vi "Main Page.vi"(8 "error in (no error)":errorcluster, 11 "Node Ptr":T1 format="%.0x") -> (0 "error out":errorcluster)   [LabVIEW 2016, in "FPGA Addon System Explorer.lvlib"]
uses:
  FPGA Addon System Explorer.lvlib
  <vilib>/NI Veristand/Custom Device API/Custom Device Item Ref.ctl
  Shared/FG Action.ctl
  <vilib>/NI/NI VeriStand Hardware Discovery/Types/Filter Type.ctl
  Shared/Constants.vi
  <vilib>/NI Veristand/Custom Device API/NI VeriStand - Get Item Property.vi
  <vilib>/NI Veristand/Custom Device API/Get Item Property (Path).vi
  <vilib>/NI Veristand/Custom Device API/Get Item Property (String).vi
  <vilib>/NI Veristand/Custom Device API/NI VeriStand - Set Item Property.vi
  <vilib>/NI Veristand/Custom Device API/Set Item Property (Path).vi
  <vilib>/NI Veristand/Custom Device API/Set Item Property (String).vi
  <vilib>/NI VeriStand/Custom Device API/Custom Device API.lvlib
  Shared/FPGA Addon Shared.lvlib
  <vilib>/NI/NI VeriStand Hardware Discovery/NIVS Hardware Discovery.lvlib
  VeriStand-FPGA-Resource-Manager/Source/FPGA Resource Manager System Definition.lvlib
panel:
  in  "RIO Browse":bool
  out "Version":string
  in  "SHDocVw.IWebBrowser":refnum<k7>(container)
  in  "RIO Device":string
  in  "Bitfile path":path
  in  "Header 2":cluster{"Section Name":string}={"Section Name"="Custom Device Item Settings"}
  in  "Header":cluster{"Section Name":string}={"Section Name"="Custom Device Item Settings"}
  in  "Description":string
  in  "Name":string
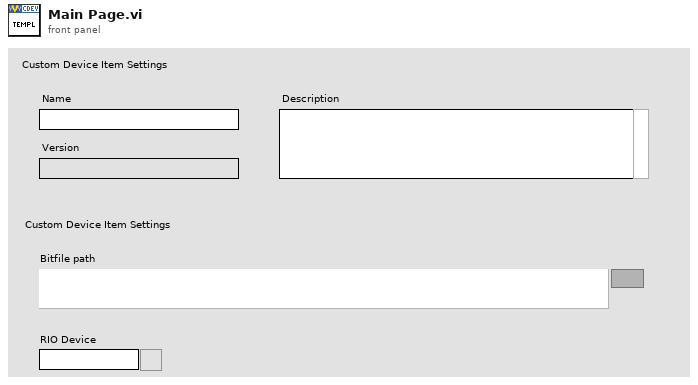
[diagram p1: front panel]
types:
  T1 = typedef "Custom Device API.lvlib/Custom Device Item Ref.ctl" = u64
  T2 = typedef "FPGA Addon Shared.lvlib/FG Action.ctl" = enum8{"GET", "SET"}
  T3 = typedef "FPGA Addon Shared.lvlib/FPGA Settings.ctl" = cluster{"Bitfile path":path, "RIO Device Address":string}
  T4 = typedef "Custom Device API.lvlib/Custom Device Item Info.ctl" = cluster{"Name":string, "Is Channel":bool, "GUID":string, "Is Waveform":bool}
  T5 = typedef "NIVS Hardware Discovery.lvlib/Filter Type.ctl" = enum16{"Device Category", "Product Name", "Ethernet", "XNET", "VISA", "FPGA", "EtherCAT Master", "DAQmx", "GPIB", "Serial"}
  T6 = typedef "Custom Device API.lvlib/Custom Device Commands.ctl" = enum16{"Default", "Item renamed", "Shutdown", "Dynamic button pressed"}
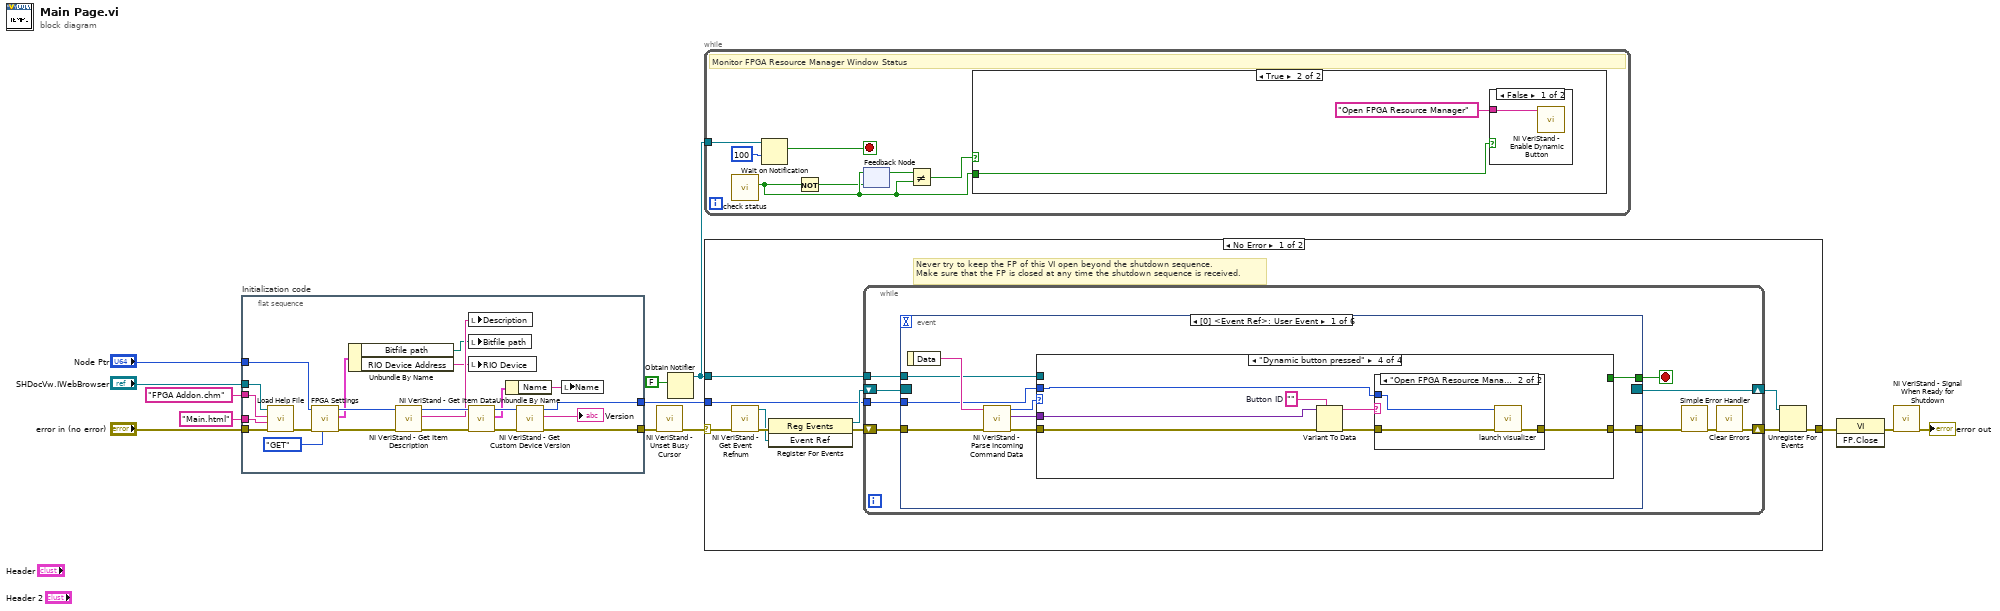
[diagram p0: block diagram]
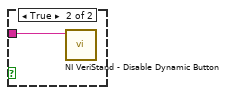
[diagram p3: hidden frame]
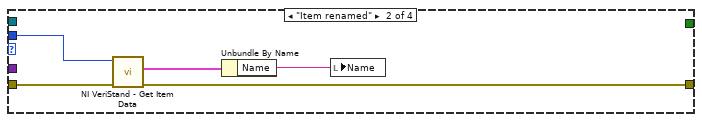
[diagram p5: hidden frame]
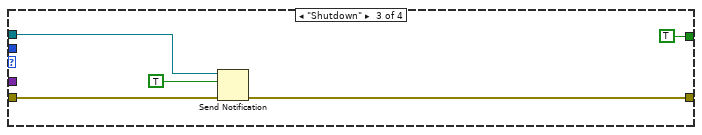
[diagram p6: hidden frame]
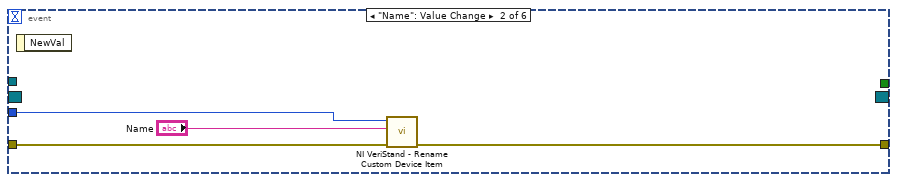
[diagram p8: hidden frame]
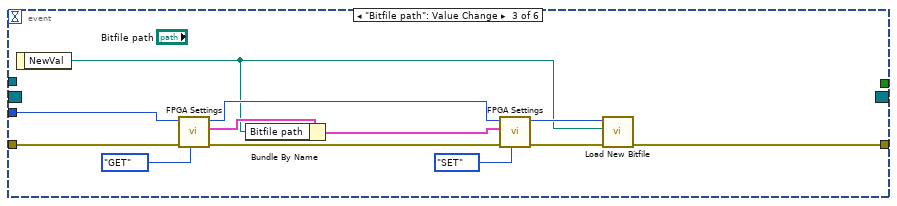
[diagram p9: hidden frame]
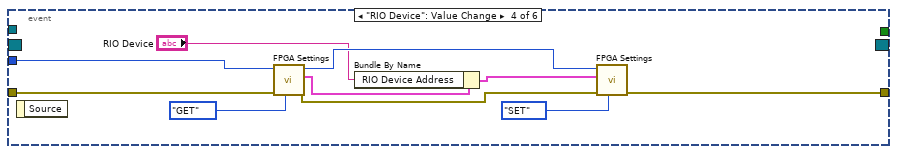
[diagram p10: hidden frame]
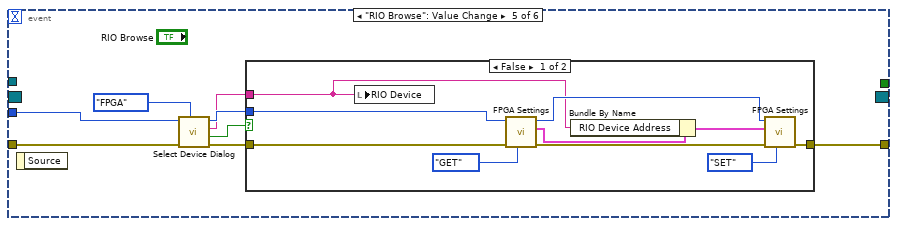
[diagram p11: hidden frame]
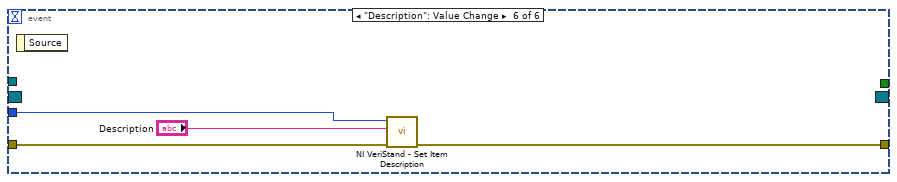
[diagram p13: hidden frame]
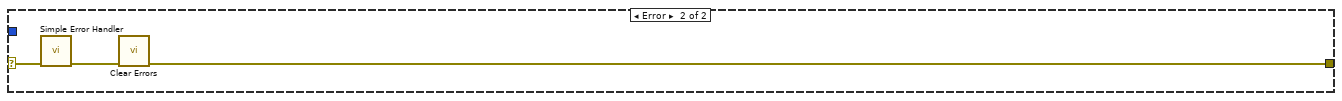
[diagram p14: hidden frame]
diagram:
  n1 = flat-sequence "Initialization code" {
    tunnel: "error in (no error)" -> [w29]
    tunnel: "Node Ptr" -> [w25]
    tunnel: [w14] -> w10
    tunnel: [w17] -> w7
    tunnel: "SHDocVw.IWebBrowser" -> [w28]
    tunnel: "Main.html" ("HTML File") -> [w27]
    tunnel: "FPGA Addon.chm" ("Main CHM File") -> [w26]
    frame #0 {
      n2 = call "Load Help File.vi"("error in (no error)"=w29, "HTML File"=w27, "Main CHM File"=w26, "SHDocVw.IWebBrowser2"=w28) -> ("error out"=w24:errorcluster)  [unwired: 7 in]
      n3 = call "FPGA Settings.vi"("Action"=FG_Action."GET", "error in (no error)"=w24, "Item Ref"=w25) -> ("error out"=w22:errorcluster, "FPGA Settings"=w20:T3, "Item Ref out"=w23:T1)  [unwired: 6 in]
      n4 = Unbundle By Name(w20) -> ("Bitfile path"=w18:path, "RIO Device Address"=w19:string)
      n5 = call <vilib>:"NI VeriStand - Get Item Description.vi"("error in (no error)"=w22, "Item Ref in"=w23) -> ("error out"=w32:errorcluster, "Description"=w33:string, "Item Ref out"=w34:T1)  [unwired: 7 out]
      n6 = local write "Description"(w33) -> ()
      n7 = local write "Bitfile path"(w18) -> ()
      n8 = local write "RIO Device"(w19) -> ()
      n9 = call <vilib>:"NI VeriStand - Get Item Data.vi"("error in (no error)"=w32, "Item Ref in"=w34) -> ("error out"=w16:errorcluster, "Item Info"=w31:T4, "Item Ref out"=w35:T1)  [unwired: 7 out]
      n10 = Unbundle By Name(w31) -> ("Name"=w30:string)
      n11 = call <vilib>:"NI VeriStand - Get Custom Device Version.vi"("error in (no error)"=w16, "Device Ref in"=w35) -> ("error out"=w14:errorcluster, "Value"=→"Version":string, "Device Ref out"=w17:T1)  [unwired: 7 in]
      n12 = local write "Name"(w30) -> ()
    }
  }
  n13 = call <vilib>:"NI VeriStand - Unset Busy Cursor.vi"("error in (no error)"=w10) -> ("error out"=w9:errorcluster)  [unwired: 10 out]
  n14 = Obtain Notifier(notification data type=FALSE) -> (notifier out=w1:refnum<notifier>)  [unwired: 3 in, 2 out]
  n15 = while {
    tunnel: w1 -> [w42]
    stop <- w41 stop-if-true
    # "Monitor FPGA Resource Manager Window Status"
    n16 = call "check status.vi"() -> ("status"=w37:bool)  [unwired: 10 in, 1 out]
    n17 = Wait on Notification(notifier=w42, timeout in ms (-1)=100) -> (notification=w41:bool)  [unwired: 2 in, 3 out]
    n18 = Not(x=w37) -> (.not. x?=w36:bool)
    n19 = feedback-in #1(w37) -> ()
    n20 = feedback #1(w36) -> (w39:bool)
    n21 = Not Equal?(x=w39, y=w37) -> (x != y?=w38:bool)
    n22 = case shown="True" w38 {
      tunnel: w37 -> [_ w43]
      frame False {
      }
      frame True {
        n23 = case shown="False" w43 {
          tunnel: "Open FPGA Resource Manager" ("Button ID") -> [w45 w46]
          frame False {
            n24 = call <vilib>:"NI VeriStand - Enable Dynamic Button.vi"("Button ID"=w45) -> ()  [unwired: 10 in, 1 out]
          }
          frame True {
            n25 = call <vilib>:"NI VeriStand - Disable Dynamic Button.vi"("Button ID"=w46) -> ()  [unwired: 10 in, 1 out]
          }
        }
      }
    }
  }
  n26 = case shown="No Error" w9 {
    selector: w9 -> [w48 w148]
    tunnel: [w53 w146] -> w13
    tunnel: w7 -> [w49 _]
    tunnel: w1 -> [w47 _]
    frame No Error {
      # "Never try to keep the FP of this VI open beyond the shutdown sequence.\nMake sure that the FP is closed at any time the shutdown sequence is received."
      n27 = call <vilib>:"NI VeriStand - Get Event Refnum.vi"("error in (no error)"=w48) -> ("error out"=w56:errorcluster, "Event Ref"=w52:refnum<user-event>)  [unwired: 9 out]
      n28 = register-events(error in=w56, w52) -> (reference out=w50:refnum<event-registration>, error out=w51:errorcluster)  [unwired: 1 in]
      n29 = while {
        tunnel: w49 -> [w61]
        shift-right: [w58] -> w54
        shift-left: w51 -> [w64]
        shift-right: [w65] -> w55
        shift-left: w50 -> [w63]
        tunnel: w47 -> [w57]
        stop <- w62 stop-if-true
        n30 = event shown="[0] <Event Ref>: User Event" {
          selector: w63 -> [_ _ _ _ _ _]
          dyn-events: [_ _ _ _ _ _] -> w65
          timeout: _ -> [_ _ _ _ _ _]
          tunnel: w64 -> [w74 w100 w107 w116 w128 w144]
          tunnel: [w70 _ _ _ _ _] -> w62
          tunnel: [w69 w99 w112 w113 w130 w143] -> w60
          tunnel: w61 -> [w68 w98 w105 w115 w129 w145]
          tunnel: w57 -> [w66 _ _ _ _ _]
          event User Event {
            n31 = event-data() -> ("Data"=w73:string)  [unwired: 1 out]
            n32 = call <vilib>:"NI VeriStand - Parse Incoming Command Data.vi"("error in (no error)"=w74, "Incoming data"=w73) -> ("error out"=w72:errorcluster, "Outgoing data"=w67:variant, "Action"=w71:T6)  [unwired: 7 out]
            n33 = case shown="\"Dynamic button pressed\"" w71 {
              tunnel: w72 -> [w75 w80 w83 w92]
              tunnel: [_ _ TRUE _] -> w70
              tunnel: [w75 w77 w82 w87] -> w69
              tunnel: w68 -> [_ w79 _ w89]
              tunnel: w67 -> [_ _ _ w91]
              tunnel: w66 -> [_ _ w84 _]
              frame "Default", Default {
              }
              frame "Item renamed" {
                n34 = call <vilib>:"NI VeriStand - Get Item Data.vi"("error in (no error)"=w80, "Item Ref in"=w79) -> ("error out"=w77:errorcluster, "Item Info"=w78:T4)  [unwired: 8 out]
                n35 = Unbundle By Name(w78) -> ("Name"=w76:string)
                n36 = local write "Name"(w76) -> ()
              }
              frame "Shutdown" {
                n37 = Send Notification(notification=TRUE, notifier=w84, error in (no error)=w83) -> (error out=w82:errorcluster)  [unwired: 1 out]
              }
              frame "Dynamic button pressed" {
                w90 = ""  # Button ID
                n38 = Variant To Data(error in=w92, type=w90, Variant=w91) -> (data=w86:string, error out=w88:errorcluster)
                n39 = case shown="\"Open FPGA Resource Manager\"" w86 {
                  tunnel: w89 -> [_ w96]
                  tunnel: w88 -> [w93 w95]
                  tunnel: [w93 w94] -> w87
                  frame "False", Default {
                  }
                  frame "Open FPGA Resource Manager" {
                    n40 = call "launch visualizer.vi"("error in (no error)"=w95, "Device Ref in"=w96) -> ("error out"=w94:errorcluster)  [unwired: 8 in, 1 out]
                  }
                }
              }
            }
          }
          event "Name": Value Change {
            n41 = event-data() -> ()  [unwired: 2 out]
            n42 = call <vilib>:"NI VeriStand - Rename Custom Device Item.vi"("error in (no error)"=w100, "New Name"="Name", "Item Ref in"=w98) -> ("error out"=w99:errorcluster)  [unwired: 1 in, 7 out]
          }
          event "Bitfile path": Value Change {
            n43 = event-data() -> ("NewVal"=w101:path)  [unwired: 1 out]
            n44 = call "FPGA Settings.vi"("Action"=FG_Action."GET", "error in (no error)"=w107, "Item Ref"=w105) -> ("error out"=w108:errorcluster, "FPGA Settings"=w103:T3, "Item Ref out"=w109:T1)  [unwired: 6 in]
            n45 = Bundle By Name(cluster=w103, "Bitfile path"=w101) -> (w102:T3)
            n46 = call "FPGA Settings.vi"("Action"=FG_Action."SET", "error in (no error)"=w108, "FPGA Settings"=w102, "Item Ref"=w109) -> ("error out"=w106:errorcluster, "Item Ref out"=w104:T1)  [unwired: 5 in, 1 out]
            n47 = call "Load New Bitfile.vi"("error in (no error)"=w106, "NewVal"=w101, "Item Ref in"=w104) -> ("error out"=w112:errorcluster)  [unwired: 7 in, 1 out]
          }
          event "RIO Device": Value Change {
            n48 = event-data() -> ()  [unwired: 2 out]
            n49 = call "FPGA Settings.vi"("Action"=FG_Action."GET", "error in (no error)"=w116, "Item Ref"=w115) -> ("error out"=w119:errorcluster, "FPGA Settings"=w118:T3, "Item Ref out"=w120:T1)  [unwired: 6 in]
            n50 = Bundle By Name(cluster=w118, "RIO Device Address"="RIO Device") -> (w117:T3)
            n51 = call "FPGA Settings.vi"("Action"=FG_Action."SET", "error in (no error)"=w119, "FPGA Settings"=w117, "Item Ref"=w120) -> ("error out"=w113:errorcluster)  [unwired: 5 in, 2 out]
          }
          event "RIO Browse": Value Change {
            n52 = event-data() -> ()  [unwired: 2 out]
            n53 = call <vilib>:"Select Device Dialog.vi"("Filter Type"=Filter_Type."FPGA", "error in (no error)"=w128, "Item Ref in"=w129) -> ("error out"=w126:errorcluster, "Cancelled?"=w125:bool, "Selected Alias"=w124:string, "Item Ref out"=w127:T1)  [unwired: 5 in]
            n54 = case shown="False" w125 {
              tunnel: w126 -> [w134 w141]
              tunnel: w127 -> [w133 _]
              tunnel: [w132 w141] -> w130
              tunnel: w124 -> [w131 _]
              frame False {
                n55 = local write "RIO Device"(w131) -> ()
                n56 = call "FPGA Settings.vi"("Action"=FG_Action."GET", "error in (no error)"=w134, "Item Ref"=w133) -> ("error out"=w137:errorcluster, "FPGA Settings"=w136:T3, "Item Ref out"=w138:T1)  [unwired: 6 in]
                n57 = Bundle By Name(cluster=w136, "RIO Device Address"=w131) -> (w135:T3)
                n58 = call "FPGA Settings.vi"("Action"=FG_Action."SET", "error in (no error)"=w137, "FPGA Settings"=w135, "Item Ref"=w138) -> ("error out"=w132:errorcluster)  [unwired: 5 in, 2 out]
              }
              frame True {
              }
            }
          }
          event "Description": Value Change {
            n59 = event-data() -> ()  [unwired: 2 out]
            n60 = call <vilib>:"NI VeriStand - Set Item Description.vi"("error in (no error)"=w144, "Description"="Description", "Item Ref in"=w145) -> ("error out"=w143:errorcluster)  [unwired: 8 out]
          }
        }
        n61 = call <vilib>:"Simple Error Handler.vi"("error in (no error)"=w60) -> ("error out"=w59:errorcluster)  [unwired: 1 in, 7 out]
        n62 = call <vilib>:"Clear Errors.vi"("error in (no error)"=w59) -> ("error out"=w58:errorcluster)  [unwired: 1 in, 5 out]
      }
      n63 = Unregister For Events(event registration refnum=w55, error in=w54) -> (error out=w53:errorcluster)
    }
    frame Error {
      n64 = call <vilib>:"Simple Error Handler.vi"("error in (no error)"=w148) -> ("error out"=w147:errorcluster)  [unwired: 1 in, 7 out]
      n65 = call <vilib>:"Clear Errors.vi"("error in (no error)"=w147) -> ("error out"=w146:errorcluster)  [unwired: 1 in, 5 out]
    }
  }
  n66 = invoke class="VI" method="FP.Close"(error in=w13) -> (error out=w12:errorcluster)  [unwired: 2 in, 2 out]
  n67 = call <vilib>:"NI VeriStand - Signal When Ready for Shutdown.vi"("error in (no error)"=w12) -> ("error out"=→"error out":errorcluster)  [unwired: 10 out]
